vi "Read u32FlagImpairmentArray.vi"(8 "error in (no error)":errorcluster, 11 "OutputToFileBasePlugin in":refnum<class "OutputToFileBasePlugin.lvclass">) -> (0 "error out":errorcluster, 2 "u32FlagImpairmentArray":T1, 3 "OutputToFileBasePlugin out":refnum<class "OutputToFileBasePlugin.lvclass">)   [LabVIEW 2014, in "OutputToFilePlugins.lvlib" / "OutputToFileBasePlugin.lvclass"]
uses:
  OutputToFileBasePlugin.lvclass
  FlagImpairPlugins/FlagImpairPluginBase_class/TypeDefs/FlagImpairmentArray.ctl
  OutputToFileBasePlugin.lvclass/OutputToFileBasePlugin.ctl
  FlagImpairPlugins/FlagImpairPluginBase_class/FlagImpairPluginBase.lvclass
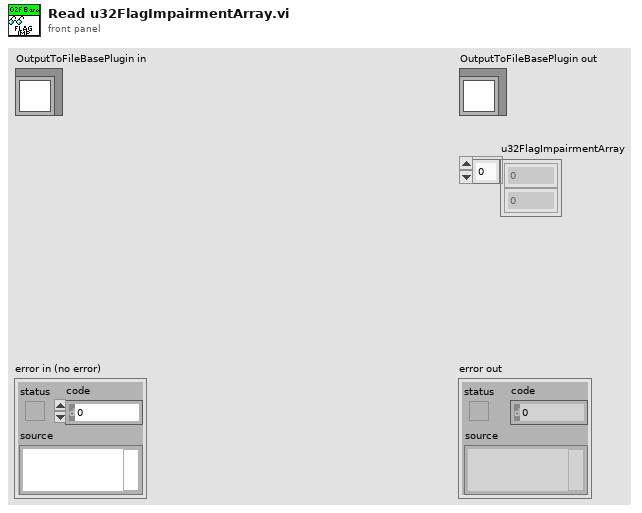
[diagram p1: front panel]
types:
  T1 = typedef "FlagImpairPlugins.lvlib/FlagImpairPluginBase.lvclass/FlagImpairmentArray.ctl" = u32[]
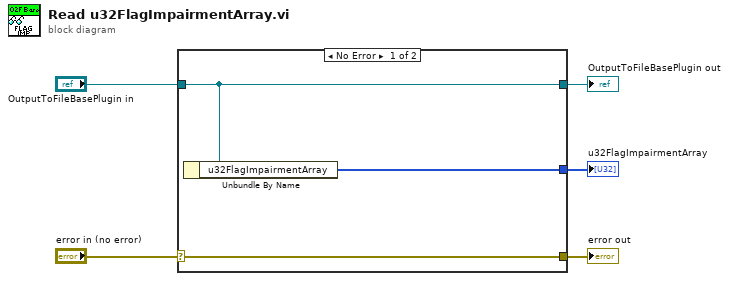
[diagram p0: block diagram]
diagram:
  n1 = case shown="No Error" "error in (no error)" {
    selector: "error in (no error)" -> [w8 w9]
    tunnel: [w8 w9] -> w4
    tunnel: [w7 w10] -> w2
    tunnel: "OutputToFileBasePlugin in" -> [w7 w10]
    tunnel: [w6 _] -> w1
    frame No Error {
      n2 = Unbundle By Name(w7) -> ("u32FlagImpairmentArray"=w6:T1)
    }
    frame Error {
    }
  }
  "error out" <- w4
  "OutputToFileBasePlugin out" <- w2
  "u32FlagImpairmentArray" <- w1
